vi "WinchEncoder.vi"(8 "error in (no error)":errorcluster, 11 "Command":T1) -> (0 "error out":errorcluster, 3 "Distance":dbl)   [LabVIEW 2013]
uses:
  EncoderCmds.ctl
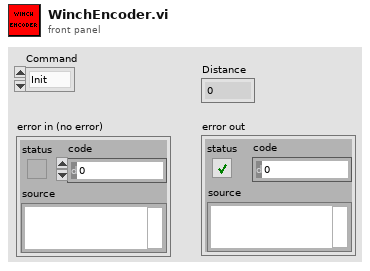
[diagram p1: front panel]
types:
  T1 = typedef "EncoderCmds.ctl" = enum16{"Init", "Reset", "Read"}
  T2 = typedef "WPI_EncoderDevRef.ctl" = cluster{"DevStatus":errorcluster, "EncoderIndex":T3, "CounterIndex":T4, "DistancePerCount":dbl, "Decoding Type":T5}
  T3 = typedef "FPGA_EncoderIdx.ctl" = enum8{"Enc 0", "Enc 1", "Enc 2", "Enc 3", "Invalid"}
  T4 = typedef "FPGA_CounterCtrSystemIndex.ctl" = enum8{"Ctr 0", "Ctr 1", "Ctr 2", "Ctr 3", "Ctr 4", "Ctr 5", "Ctr 6", "Ctr 7", "Invalid"}
  T5 = typedef "WPI_EncoderType.ctl" = enum16{"1x", "2x", "4x"}
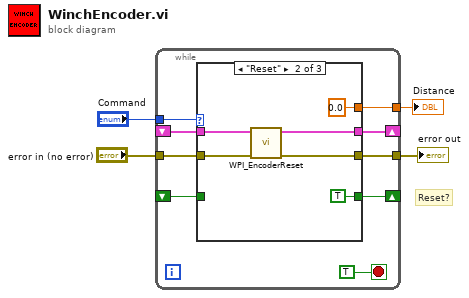
[diagram p0: block diagram]
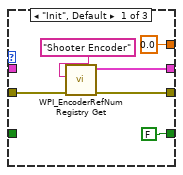
[diagram p2: hidden frame]
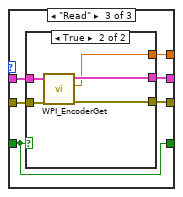
[diagram p3: hidden frame]
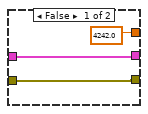
[diagram p4: hidden frame]
diagram:
  # "Reset?"
  n1 = while {
    tunnel: "Command" -> [w13]
    shift-right: [w11] -> _
    shift-left: _ -> [w7]
    shift-right: [w10] -> _
    shift-left: _ -> [w6]
    tunnel: "error in (no error)" -> [w9]
    tunnel: [w8] -> w3
    tunnel: [w5] -> w4
    stop <- TRUE stop-if-true
    n2 = case shown="\"Reset\"" w13 {
      tunnel: [w18 w22 w29] -> w11
      tunnel: [FALSE TRUE w26] -> w10
      tunnel: w9 -> [w16 w24 w30]
      tunnel: [w15 w23 w28] -> w8
      tunnel: w7 -> [_ w25 w31]
      tunnel: w6 -> [_ _ w26]
      tunnel: [0.0 ("Distance") 0.0 ("Distance") w27] -> w5
      frame "Init", Default {
        n3 = call <vilib>:"WPI_EncoderRefNum Registry Get.vi"("error in (no error)"=w16, "refnum name"="Shooter Encoder") -> ("error out"=w15:errorcluster, "EncoderDevRef"=w18:T2)  [unwired: 8 in]
      }
      frame "Reset" {
        n4 = call <vilib>:"WPI_EncoderReset.vi"("error in (no error)"=w24, "EncoderDevRef"=w25) -> ("error out"=w23:errorcluster, "EncoderDevRef"=w22:T2)  [unwired: 8 in]
      }
      frame "Read" {
        n5 = case shown="True" w26 {
          tunnel: w31 -> [w34 w39]
          tunnel: w30 -> [w32 w38]
          tunnel: [w34 w37] -> w29
          tunnel: [w32 w36] -> w28
          tunnel: [4242.0 ("Distance") w35] -> w27
          frame False {
          }
          frame True {
            n6 = call <vilib>:"WPI_EncoderGet.vi"("error in (no error)"=w38, "EncoderDevRef"=w39) -> ("error out"=w36:errorcluster, "Distance"=w35:dbl, "EncoderDevRef"=w37:T2)  [unwired: 4 in, 3 out]
          }
        }
      }
    }
  }
  "error out" <- w3
  "Distance" <- w4
